vi "Write Channel.vi"(8 "error in (no error)":errorcluster, 9 "Channel List(\"\")":string, 10 "Value (0)":dbl, 11 "VISA resource name":refnum<visa-resource-name>) -> (0 "error out":errorcluster, 3 "VISA resource name out":refnum<visa-resource-name>)   [LabVIEW 2015, in "Keithley DMM6500 DAQ6500 Series.lvlib"]
doc: "Writes a value to a channel.\nFor a channel with a power state of OFF, an error is generated. No action is taken on any channel in the specified channel list.\nFor DAC channels, the value is expected to be the set floating-point voltage or current. Also, an error is generated if the value is out of range. No action is taken on any channel in the specified channel list.\nFor digital I/O channels, the value becomes the settings of the digital output.\nFor totalizer channels, you can send 0 to reset the totalizer channel to 0."
uses:
  <instrlib>/Keithley DMM6500 DAQ6500 Series/Keithley DMM6500 DAQ6500 Series.lvlib
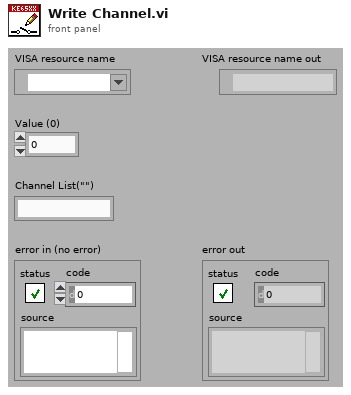
[diagram p1: front panel]
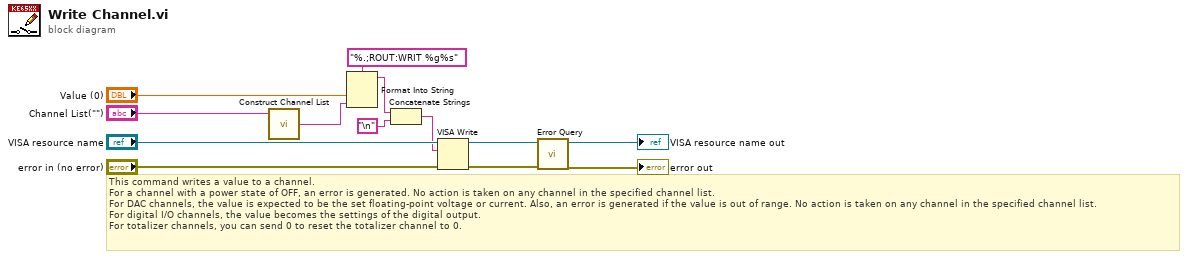
[diagram p0: block diagram]
diagram:
  # "This command writes a value to a channel.\nFor a channel with a power state of OFF, an error is generated. No action is taken on any channel in the specified channel list.\nFor DAC channels, the value is expected to be the set floating-point voltage or current. Also, an error is generated if the value is out of range. No action is taken on any channel in the specified channel list.\nFor digital I/O channels, the value becomes the settings of the digital output.\nFor totalizer channels, you can send 0 to reset the totalizer channel to 0."
  n1 = call <instrlib>:"Construct Channel List.vi"("Channel List"="Channel List(\"\")") -> ("Channel List String"=w2:string)  [unwired: 2 in]
  n2 = Format Into String(format string="%.;ROUT:WRIT %g%s", "Value (0)", w2) -> (resulting string=w5:string)  [unwired: 2 in, 1 out]
  n3 = Concatenate Strings(w5, "\n") -> (w6:string)
  n4 = VISA Write(VISA resource name="VISA resource name", write buffer=w6, error in (no error)="error in (no error)") -> (VISA resource name out=w10:refnum<visa-resource-name>, error out=w9:errorcluster)  [unwired: 1 out]
  n5 = call <instrlib>:"Error Query.vi"("error in (no error)"=w9, "VISA resource name"=w10) -> ("error out"=→"error out":errorcluster, "VISA resource name out"=→"VISA resource name out":refnum<visa-resource-name>)  [unwired: 6 in, 2 out]
